vi "to_item.vi"(8 "error in (no error)":errorcluster, 11 "Table in":refnum<class "Table.lvclass">) -> (0 "error out":errorcluster, 3 "Item out":refnum<class "Item.lvclass">)   [LabVIEW 2020, in "toml_edit.lvlib" / "Table.lvclass"]
uses:
  Table.lvclass
  Item/Item.lvclass
  Table.lvclass/Table.ctl
  dragon_toml_64.dll
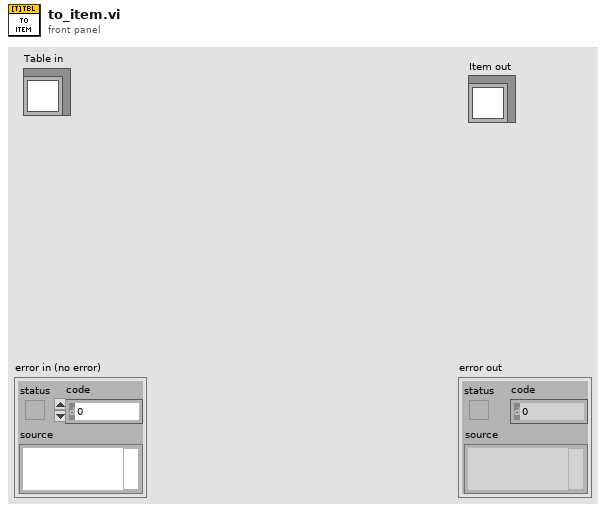
[diagram p1: front panel]
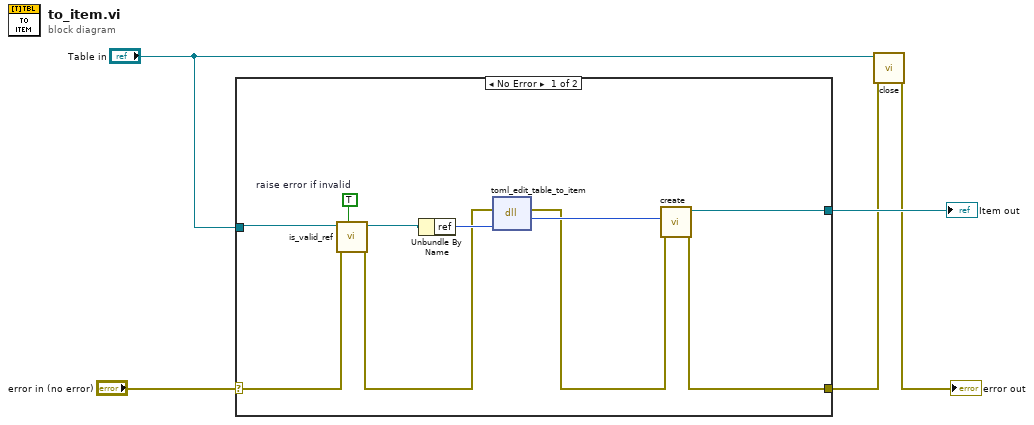
[diagram p0: block diagram]
diagram:
  n1 = case shown="No Error" "error in (no error)" {
    selector: "error in (no error)" -> [w7 w16]
    tunnel: [w11 w16] -> w1
    tunnel: "Table in" -> [w8 _]
    tunnel: [w13 _] -> w3
    frame No Error {
      w10 = TRUE  # raise error if invalid
      n2 = call-dynamic "is_valid_ref.vi"("raise error if invalid? (False)"=w10, "error in (no error)"=w7, "Table in"=w8) -> ("error out"=w6:errorcluster, "Table out"=w9:refnum<class "Table.lvclass">)  [unwired: 6 in, 1 out]
      n3 = Unbundle By Name(w9) -> ("ref"=w15:u64)
      n4 = dll-call lib="C:/Projects/labview-project-load-tools/source/submodules/toml-edit-labview/lv_src/dragon_toml_*.*" fn="toml_edit_table_to_item"(error in=w6, "table_ref"=w15) -> (error out=w12:errorcluster, "item_ref"=w14:u64)  [unwired: 3 in, 1 out]
      n5 = call "create.vi"("error in (no error)"=w12, "ref"=w14) -> ("error out"=w11:errorcluster, "Item out"=w13:refnum<class "Item.lvclass">)  [unwired: 7 in, 1 out]
    }
    frame Error {
    }
  }
  "Item out" <- w3
  n6 = call "close.vi"("error in (no error)"=w1, "Table in"="Table in") -> ("error out"=→"error out":errorcluster)  [unwired: 9 in]
